vi "neo_tmp.vi"() -> ()   [LabVIEW 2012]
uses:
  E:/Kinect/Neobotix/CSInterface/RosBridgeDotNet.dll
  RosBridgeDotNet.dll
panel:
  out "container2":dbl[](graph)
  in  "MelyIP":u16(ring) items=["192.168.0.152", "127.0.0.1"]
  in  "gear":i32(knob)=12 scale=20.0..5.0
  in  "0seb":bool
  in  "Jobb":dbl(slide) scale=-2.0..2.0
  in  "Bal":dbl(slide) scale=-2.0..2.0 scale format="%0#1_1g"
  out "Joy":picture
  in  "Disconn":bool
  out "IPEredmeny":T1(array[cluster]) {"Status" items=["Success"=0, "DestinationNetworkUnreachable"=11002, "DestinationHostUnreachable"=11003, "DestinationProhibited, DestinationProtocolUnreachable"=11004, "DestinationPortUnreachable"=11005, "NoResources"=11006, "BadOption"=11007, "HardwareError"=11008, "PacketTooBig"=11009, "TimedOut"=11010, "BadRoute"=11012, "TtlExpired"=11013, "TtlReassemblyTimeExceeded"=11014, "ParameterProblem"=11015, "SourceQuench"=11016, "BadDestination"=11018, "DestinationUnreachable"=11040, "TimeExceeded"=11041, "BadHeader"=11042, "UnrecognizedNextHeader"=11043, "IcmpError"=11044, "DestinationScopeMismatch"=11045, "Unknown"=-1]}
  in  "Ping":bool
  in  "MessN":bool
  out "Error Out":errorcluster
  in  "Connnect":bool
  out "Connected":bool
  in  "Stop Button":bool
  out "container1":dbl[](graph)
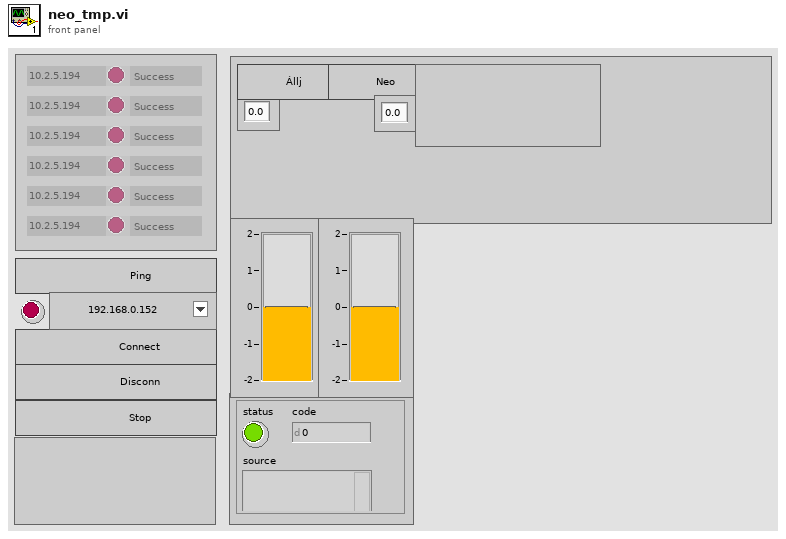
[diagram p1: front panel]
types:
  T1 = cluster{"pingelhet":bool, "IpAddress":string, "Status":i32}[]
  T2 = cluster{"Width":u16, "Style":enum32{"Solid", "Dash", "Dot", "DashDot", "DashDotDot"}}
  T3 = cluster{"left":i16, "top":i16, "right":i16, "bottom":i16}
  T4 = cluster{"pingelhet":bool, "IpAddress":string, "Status":i32}
  T5 = typedef "LVMouseTypeDef.ctl" = cluster{"Mouse Position":cluster{"X":i32, "Y":i32}, "Mouse Modifiers":cluster{"Button Down":bool, "Shift Mod":bool, "Menu Mod":bool, "Option Mod":bool}}
  T6 = typedef "LVBoundsTypeDef.ctl" = cluster{"Width":u32, "Height":u32}
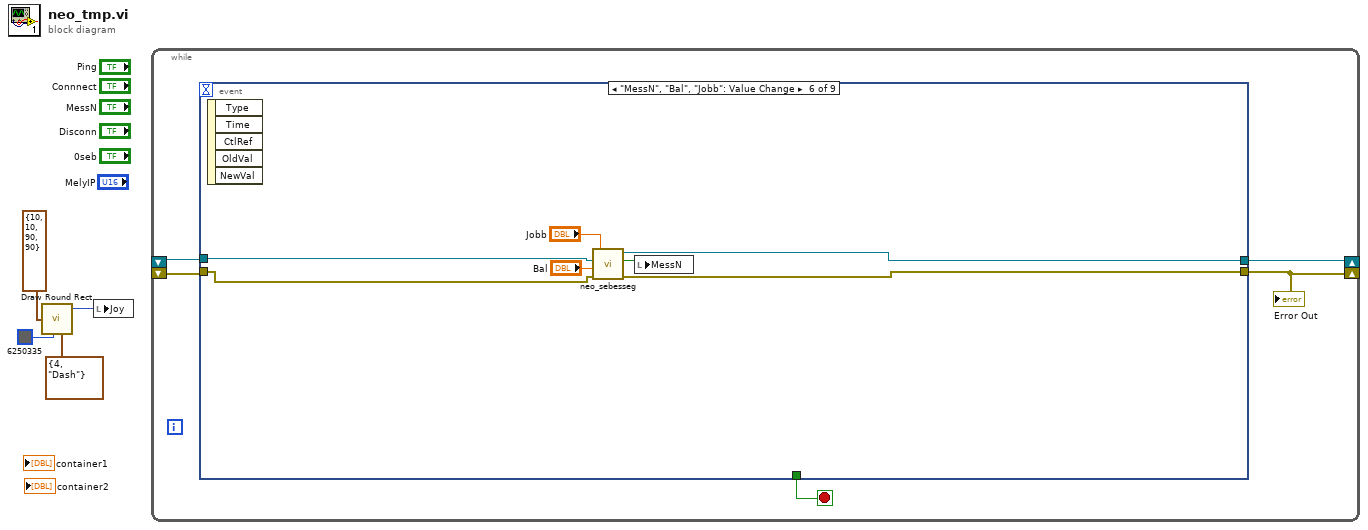
[diagram p0: block diagram]
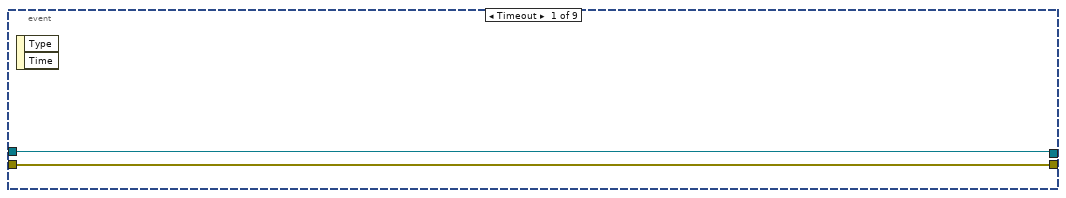
[diagram p2: hidden frame]
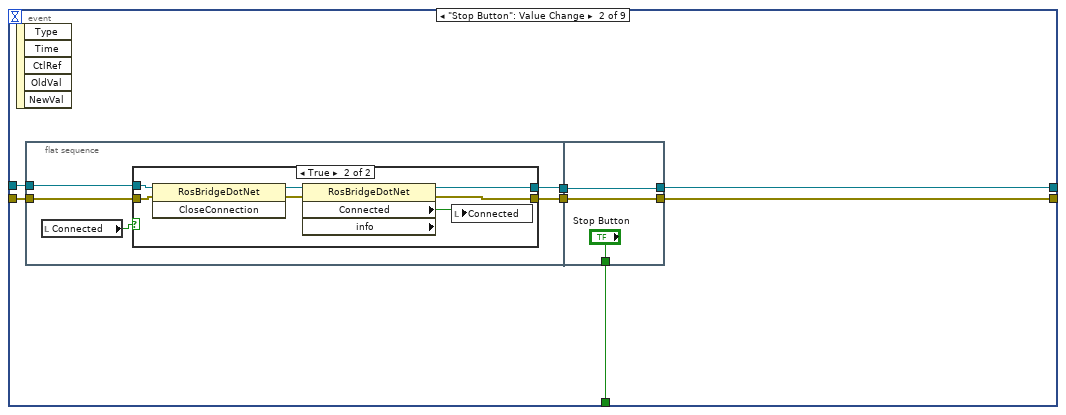
[diagram p3: hidden frame]
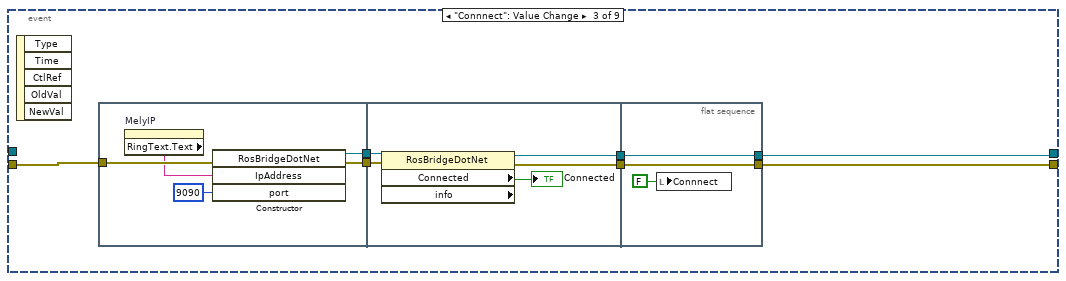
[diagram p5: hidden frame]
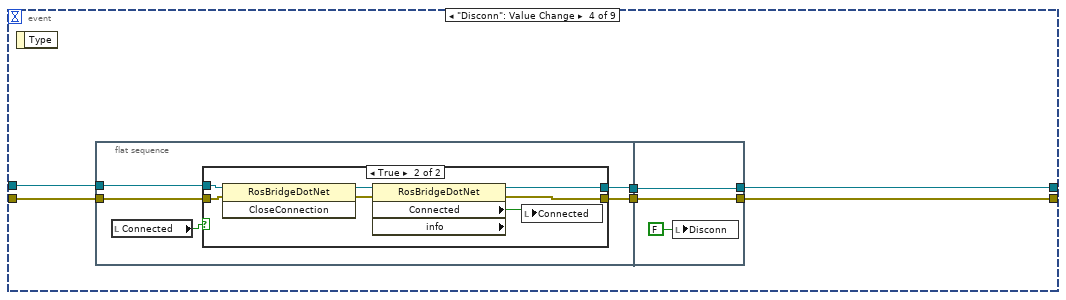
[diagram p6: hidden frame]
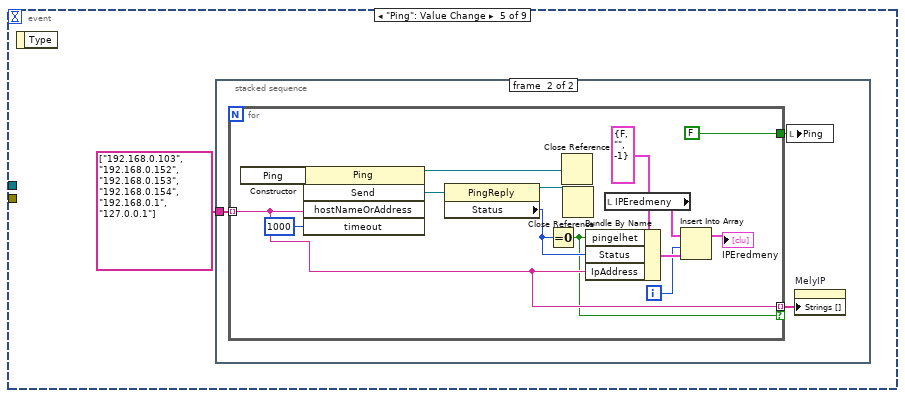
[diagram p8: hidden frame]
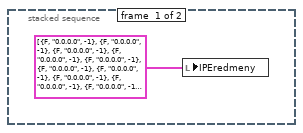
[diagram p9: hidden frame]
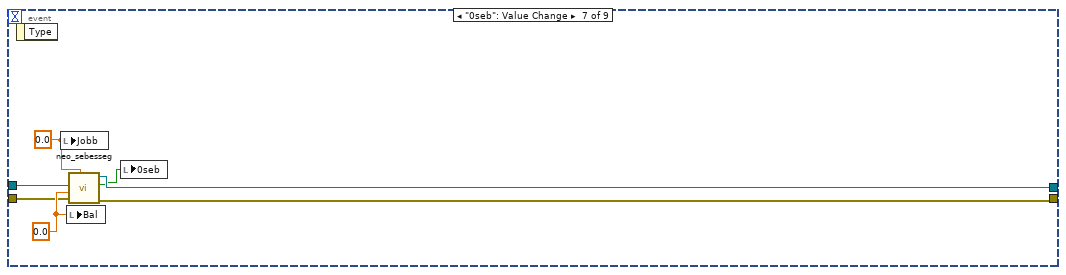
[diagram p10: hidden frame]
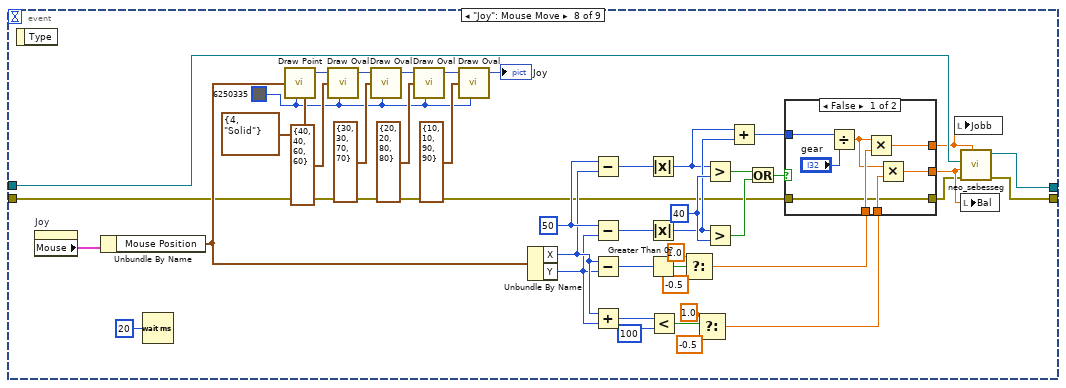
[diagram p11: hidden frame]
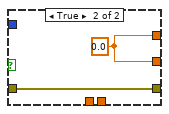
[diagram p12: hidden frame]
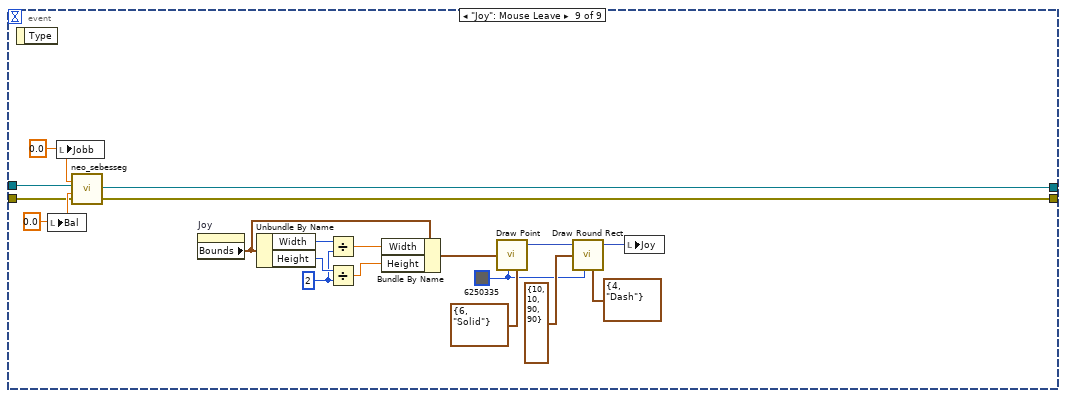
[diagram p13: hidden frame]
diagram:
  n1 = call <vilib>:"Draw Round Rect.vi"("rect"=T3 {"left"=10, "top"=10, "right"=90, "bottom"=90}, "color(black)"=u32 6250335, "pen"=T2 {"Width"=4, "Style"=enum."Dash"}) -> ("new picture"=w1:picture)  [unwired: 6 in]
  n2 = local write "Joy"(w1) -> ()
  n3 = while {
    shift-right: [w8] -> _
    shift-left: _ -> [w6]
    shift-right: [w5] -> _
    shift-left: _ -> [w7]
    stop <- w9 stop-if-true
    n4 = event shown="[5] \"MessN\", \"Bal\", \"Jobb\": Value Change" {
      selector: _ -> [_ _ _ _ _ _ _ _ _]
      dyn-events: _ -> [_ _ _ _ _ _ _ _ _]
      timeout: _ -> [_ _ _ _ _ _ _ _ _]
      tunnel: [_ w12 _ _ _ _ _ _ _] -> w9
      tunnel: [w11 w16 w36 w57 _ w102 w110 w145 w179] -> w8
      tunnel: [w10 w15 w37 w56 _ w101 w106 w146 w180] -> w5
      tunnel: w7 -> [w10 w17 w42 w58 _ w103 w107 w113 w181]
      tunnel: w6 -> [w11 w18 _ w59 _ w104 w111 w147 w182]
      event Timeout {
        n5 = event-data() -> ()  [unwired: 1 in, 2 out]
      }
      event "Stop Button": Value Change {
        n6 = event-data() -> ()  [unwired: 1 in, 5 out]
        n7 = flat-sequence {
          tunnel: w18 -> [w23]
          tunnel: w17 -> [w22]
          tunnel: [w21] -> w14
          tunnel: [w20] -> w13
          tunnel: [w34] -> w15
          tunnel: [w35] -> w16
          tunnel: w14 -> [w35]
          tunnel: w13 -> [w34]
          tunnel: ["Stop Button"] -> w12
          frame #0 {
            n8 = local read "Connected"() -> (w19:bool)
            n9 = case shown="True" w19 {
              tunnel: w23 -> [w25 w30]
              tunnel: w22 -> [w24 w29]
              tunnel: [w25 w28] -> w21
              tunnel: [w24 w27] -> w20
              frame False {
              }
              frame True {
                n10 = invoke class="RosBridgeDotNet" method="CloseConnection"(reference=w30, error in=w29) -> (reference out=w31:refnum<k24>, error out=w32:errorcluster)  [unwired: 1 in, 1 out]
                n11 = property class="RosBridgeDotNet" props=["Connected", "info"](reference=w31, error in=w32) -> (reference out=w28:refnum<k24>, error out=w27:errorcluster, "Connected"=w26:bool)  [unwired: 1 out]
                n12 = local write "Connected"(w26) -> ()
              }
            }
          }
          frame #1 {
          }
        }
      }
      event "Connnect": Value Change {
        n13 = event-data() -> ()  [unwired: 1 in, 5 out]
        n14 = flat-sequence {
          tunnel: [w46] -> w41
          tunnel: [w45] -> w40
          tunnel: w42 -> [w44]
          tunnel: w41 -> [w51]
          tunnel: w40 -> [w50]
          tunnel: [w49] -> w39
          tunnel: [w48] -> w38
          tunnel: w39 -> [w53]
          tunnel: w38 -> [w54]
          tunnel: [w54] -> w37
          tunnel: [w53] -> w36
          frame #0 {
            n15 = property on="MelyIP" class="Ring (strict)"() -> ("RingText.Text"=w43:string)  [unwired: 2 in, 2 out]
            n16 = constructor class="RosBridgeDotNet"(error in=w44, "IpAddress"=w43, "port"=9090) -> (reference out=w46:refnum<k24>, error out=w45:errorcluster)  [unwired: 2 in, 3 out]
          }
          frame #1 {
            n17 = property class="RosBridgeDotNet" props=["Connected", "info"](reference=w51, error in=w50) -> (reference out=w49:refnum<k24>, error out=w48:errorcluster, "Connected"=→"Connected":bool)  [unwired: 1 out]
          }
          frame #2 {
            n18 = local write "Connnect"(FALSE ("Connnect")) -> ()
          }
        }
      }
      event "Disconn": Value Change {
        n19 = event-data() -> ()  [unwired: 1 in, 1 out]
        n20 = flat-sequence {
          tunnel: w59 -> [w66]
          tunnel: w58 -> [w65]
          tunnel: [w64] -> w61
          tunnel: [w63] -> w60
          tunnel: [w77] -> w56
          tunnel: [w78] -> w57
          tunnel: w61 -> [w78]
          tunnel: w60 -> [w77]
          frame #0 {
            n21 = local read "Connected"() -> (w62:bool)
            n22 = case shown="True" w62 {
              tunnel: w66 -> [w68 w73]
              tunnel: w65 -> [w67 w72]
              tunnel: [w68 w71] -> w64
              tunnel: [w67 w70] -> w63
              frame False {
              }
              frame True {
                n23 = invoke class="RosBridgeDotNet" method="CloseConnection"(reference=w73, error in=w72) -> (reference out=w74:refnum<k24>, error out=w75:errorcluster)  [unwired: 1 in, 1 out]
                n24 = property class="RosBridgeDotNet" props=["Connected", "info"](reference=w74, error in=w75) -> (reference out=w71:refnum<k24>, error out=w70:errorcluster, "Connected"=w69:bool)  [unwired: 1 out]
                n25 = local write "Connected"(w69) -> ()
              }
            }
          }
          frame #1 {
            n26 = local write "Disconn"(FALSE ("Disconn")) -> ()
          }
        }
      }
      event "Ping": Value Change {
        n27 = event-data() -> ()  [unwired: 1 in, 1 out]
        n28 = stacked-sequence {
          tunnel: string[] ["192.168.0.103", "192.168.0.152", "192.168.0.153", "192.168.0.154", "192.168.0.1", "127.0.0.1"] ("IPCimek 3") -> [_ w82]
          frame #0 {
            n29 = local write "IPEredmeny"(T1 [{"pingelhet"=FALSE, "IpAddress"="0.0.0.0", "Status"=-1}, {"pingelhet"=FALSE, "IpAddress"="0.0.0.0", "Status"=-1}, {"pingelhet"=FALSE, "IpAddress"="0.0.0.0", "Status"=-1}, {"pingelhet"=FALSE, "IpAddress"="0.0.0.0", "Status"=-1}, {"pingelhet"=FALSE, "IpAddress"="0.0.0.0", "Status"=-1}, {"pingelhet"=FALSE, "IpAddress"="0.0.0.0", "Status"=-1}, {"pingelhet"=FALSE, "IpAddress"="0.0.0.0", "Status"=-1}, {"pingelhet"=FALSE, "IpAddress"="0.0.0.0", "Status"=-1}, {"pingelhet"=FALSE, "IpAddress"="0.0.0.0", "Status"=-1}, {"pingelhet"=FALSE, "IpAddress"="0.0.0.0", "Status"=-1}, {"pingelhet"=FALSE, "IpAddress"="0.0.0.0", "Status"=-1}] ("IPEredmeny 2")) -> ()
          }
          frame #1 {
            n30 = for {
              tunnel: [FALSE ("Ping")] -> w83
              tunnel: w82 -> [w85] mode=indexing
              tunnel: [w85] -> w81 mode=indexing if=w84
              i -> [w89]
              n31 = constructor class="Ping"() -> (reference out=w96:refnum<k24>)  [unwired: 3 in, 2 out]
              n32 = invoke class="Ping" method="Send"(reference=w96, "hostNameOrAddress"=w85, "timeout"=1000) -> (reference out=w94:refnum<k24>, "Send"=w97:refnum<k24>)  [unwired: 2 in, 3 out]
              n33 = property class="PingReply"(reference=w97) -> (reference out=w95:refnum<k24>, "Status"=w92:i32)  [unwired: 1 in, 1 out]
              n34 = Equal To 0?(x=w92) -> (x = 0?=w84:bool)
              n35 = Close Reference(reference=w94) -> ()  [unwired: 1 in, 1 out]
              n36 = Close Reference(reference=w95) -> ()  [unwired: 1 in, 1 out]
              n37 = Bundle By Name(cluster=T4 {"pingelhet"=FALSE, "IpAddress"="", "Status"=-1} ("element"), "pingelhet"=w84, "Status"=w92, "IpAddress"=w85) -> (w90:T4)
              n38 = local read "IPEredmeny"() -> (w86:T1)
              n39 = Insert Into Array(array=w86, index=w89, new element=w90) -> (→"IPEredmeny":T1)
            }
            n40 = local write "Ping"(w83) -> ()
            n41 = property on="MelyIP" class="Ring (strict)"("Strings []"=w81) -> ()  [unwired: 2 in, 2 out]
          }
        }
      }
      event "MessN", "Bal", "Jobb": Value Change {
        n42 = event-data() -> ()  [unwired: 1 in, 5 out]
        n43 = call "neo_sebesseg.vi"("Jobb"="Jobb", "error in (no error)"=w103, "Bal"="Bal", "new reference in"=w104) -> ("error out"=w101:errorcluster, "vissza"=w98:bool, ".NET Refnum out"=w102:refnum<k24>)  [unwired: 5 in]
        n44 = local write "MessN"(w98) -> ()
      }
      event "0seb": Value Change {
        w109 = 0.0 ("element")
        w108 = 0.0 ("element")
        n45 = event-data() -> ()  [unwired: 1 in, 1 out]
        n46 = local write "Jobb"(w109) -> ()
        n47 = local write "Bal"(w108) -> ()
        n48 = call "neo_sebesseg.vi"("Jobb"=w109, "error in (no error)"=w107, "Bal"=w108, "new reference in"=w111) -> ("error out"=w106:errorcluster, "vissza"=w105:bool, ".NET Refnum out"=w110:refnum<k24>)  [unwired: 5 in]
        n49 = local write "0seb"(w105) -> ()
      }
      event "Joy": Mouse Move {
        w114 = u32 6250335
        w138 = 40 ("y")
        w139 = 50
        n50 = event-data() -> ()  [unwired: 1 in, 1 out]
        n51 = property on="Joy" class="Pict"() -> ("Mouse"=w155:T5)  [unwired: 2 in, 2 out]
        n52 = Unbundle By Name(w155) -> ("Mouse Position"=w141:cluster{"X":i32, "Y":i32})
        n53 = Wait (ms)(milliseconds to wait=u32 20) -> ()  [unwired: 1 out]
        n54 = call <vilib>:"Draw Point.vi"("point(x,y)"=w141, "color(black)"=w114, "pen"=T2 {"Width"=4, "Style"=enum."Solid"}) -> ("new picture"=w151:picture)  [unwired: 6 in]
        n55 = call <vilib>:"Draw Oval.vi"("picture"=w151, "rect"=T3 {"left"=40, "top"=40, "right"=60, "bottom"=60}, "color(black)"=w114) -> ("new picture"=w153:picture)  [unwired: 6 in]
        n56 = call <vilib>:"Draw Oval.vi"("picture"=w153, "rect"=T3 {"left"=30, "top"=30, "right"=70, "bottom"=70}, "color(black)"=w114) -> ("new picture"=w149:picture)  [unwired: 6 in]
        n57 = call <vilib>:"Draw Oval.vi"("picture"=w149, "rect"=T3 {"left"=20, "top"=20, "right"=80, "bottom"=80}, "color(black)"=w114) -> ("new picture"=w143:picture)  [unwired: 6 in]
        n58 = call <vilib>:"Draw Oval.vi"("picture"=w143, "rect"=T3 {"left"=10, "top"=10, "right"=90, "bottom"=90}, "color(black)"=w114) -> ("new picture"=→"Joy":picture)  [unwired: 6 in]
        n59 = Unbundle By Name(w141) -> ("X"=w132:i32, "Y"=w131:i32)
        n60 = Subtract(x=w139, y=w132) -> (x-y=w128:i32)
        n61 = Subtract(x=w139, y=w131) -> (x-y=w127:i32)
        n62 = Subtract(x=w132, y=w131) -> (x-y=w133:i32)
        n63 = Add(x=w132, y=w131) -> (x+y=w130:i32)
        n64 = Absolute Value(x=w128) -> (abs(x)=w117:i32)
        n65 = Absolute Value(x=w127) -> (abs(x)=w118:i32)
        n66 = Greater Than 0?(x=w133) -> (x > 0?=w126:bool)
        n67 = Less?(x=w130, y=100) -> (x < y?=w121:bool)
        n68 = Select(t=1.0, s=w126, f=-0.5) -> (s? t:f=w123:dbl)
        n69 = Select(t=1.0, s=w121, f=-0.5) -> (s? t:f=w119:dbl)
        n70 = Greater?(x=w117, y=w138) -> (0:w136:bool)
        n71 = Greater?(x=w118, y=w138) -> (0:w137:bool)
        n72 = Add(x=w117, y=w118) -> (x+y=w116:i32)
        n73 = Or(x=w136, y=w137) -> (x .or. y?=w140:bool)
        n74 = case shown="False" w140 {
          tunnel: [w162 w165] -> w134
          tunnel: [w159 w165] -> w135
          tunnel: w116 -> [w163 _]
          tunnel: w123 -> [w161 _]
          tunnel: w119 -> [w160 _]
          tunnel: w113 -> [w156 w164]
          tunnel: [w156 w164] -> w112
          frame False {
            n75 = Divide(x=w163, y="gear") -> (x/y=w158:dbl)
            n76 = Multiply(x=w158, y=w161) -> (x*y=w162:dbl)
            n77 = Multiply(x=w158, y=w160) -> (x*y=w159:dbl)
          }
          frame True {
            w165 = 0.0 ("Jobb")
          }
        }
        n78 = local write "Jobb"(w134) -> ()
        n79 = call "neo_sebesseg.vi"("Jobb"=w134, "error in (no error)"=w112, "Bal"=w135, "new reference in"=w147) -> ("error out"=w146:errorcluster, ".NET Refnum out"=w145:refnum<k24>)  [unwired: 5 in, 1 out]
        n80 = local write "Bal"(w135) -> ()
      }
      event "Joy": Mouse Leave {
        w166 = u32 6250335
        w176 = u32 2 ("y")
        w184 = 0.0 ("element")
        w183 = 0.0 ("element")
        n81 = event-data() -> ()  [unwired: 1 in, 1 out]
        n82 = local write "Bal"(w183) -> ()
        n83 = local write "Jobb"(w184) -> ()
        n84 = call "neo_sebesseg.vi"("Jobb"=w184, "error in (no error)"=w181, "Bal"=w183, "new reference in"=w182) -> ("error out"=w180:errorcluster, ".NET Refnum out"=w179:refnum<k24>)  [unwired: 5 in, 1 out]
        n85 = property on="Joy" class="Pict"() -> ("Bounds"=w174:T6)  [unwired: 2 in, 2 out]
        n86 = Unbundle By Name(w174) -> ("Width"=w178:u32, "Height"=w177:u32)
        n87 = Divide(x=w178, y=w176) -> (x/y=w175:dbl)
        n88 = Divide(x=w177, y=w176) -> (x/y=w173:dbl)
        n89 = Bundle By Name(cluster=w174, "Width"=w175, "Height"=w173) -> (w171:T6)
        n90 = call <vilib>:"Draw Point.vi"("point(x,y)"=w171, "color(black)"=w166, "pen"=T2 {"Width"=6, "Style"=enum."Solid"}) -> ("new picture"=w170:picture)  [unwired: 6 in]
        n91 = call <vilib>:"Draw Round Rect.vi"("picture"=w170, "rect"=T3 {"left"=10, "top"=10, "right"=90, "bottom"=90}, "color(black)"=w166, "pen"=T2 {"Width"=4, "Style"=enum."Dash"}) -> ("new picture"=w169:picture)  [unwired: 5 in]
        n92 = local write "Joy"(w169) -> ()
      }
    }
    "Error Out" <- w5
  }
